vi "Init.vi"(8 "error in (no error)":errorcluster, 10 "Address":string, 11 "ArduinoTranslationStage in":refnum<class "ArduinoTranslationStage.lvclass">) -> (0 "error out":errorcluster, 3 "ArduinoTranslationStage out":refnum<class "ArduinoTranslationStage.lvclass">)   [LabVIEW 2023, in "ArduinoTranslationStage.lvlib" / "ArduinoTranslationStage.lvclass"]
uses:
  ArduinoTranslationStage.lvclass
  ArduinoTranslationStage.lvclass/ArduinoTranslationStage.ctl
  <vilib>/Instr/_visa.llb/Select Event Type.ctl
  Interfaces/InitDeinitInterface/InitDeinitComm Messages/InitDone Msg/InitDone Msg.lvclass
  <vilib>/ActorFramework/Actor/Actor.lvclass
  typedefs/instrumentType.ctl
  typedefs/typedefs.lvlib
  Applications/National Instruments/LabVIEW 2023 64-bit/vi.lib/ActorFramework/Actor/Actor.lvclass
  Users/alexandrosspiliotis/Documents/LV_DAQ_Project/UIs/ArduinoTranslationStageUI/ArduinoTranslationStageActor/ArduinoTranslationStage Actor/ArduinoTranslationStage.lvclass
  Users/alexandrosspiliotis/Documents/LV_DAQ_Project/Interfaces/InitDeinitInterface/InitDeinit/InitDeinit.lvclass
  Users/alexandrosspiliotis/Documents/LV_DAQ_Project/Interfaces/AbstractInstrumentClasses/StepperMotorControllers_LV/StepperMotorController/StepperMotorController.lvclass
  Users/alexandrosspiliotis/Documents/LV_DAQ_Project/Interfaces/AbstractInstrumentClasses/TranslationStages_LV/TranslationStageInterface/TranslationStagesInterface.lvclass
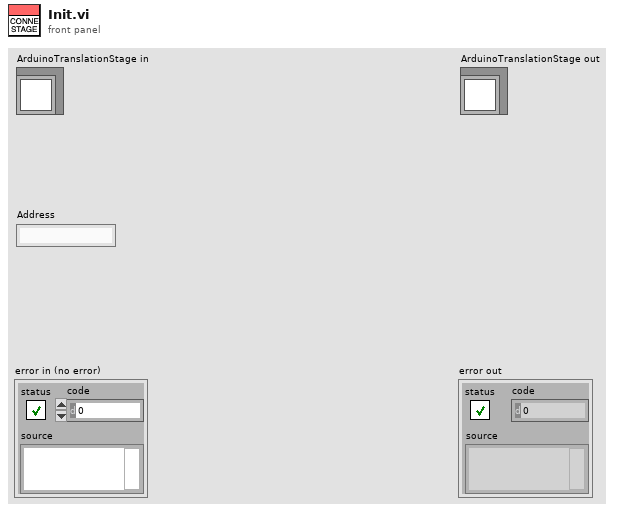
[diagram p1: front panel]
types:
  T1 = typedef "typedefs.lvlib/instrumentType.ctl" = enum16{"Spectrometer", "Camera", "Stepper"}
  T2 = typedef "Select Event Type.ctl" = u32
  T3 = typedef "typedefs.lvlib/InstrumentData.ctl" = cluster{"Instr Error":errorcluster, "Address":cluster{"address type":enum16{"VISA", "Index"}, "Address":string, "instrument type":T1}, "CurrentState":cluster{"Initialized":bool, "Connected":bool, "Running":bool, "Error":bool}, "Enqueuer":refnum<class "Message Enqueuer.lvclass">}
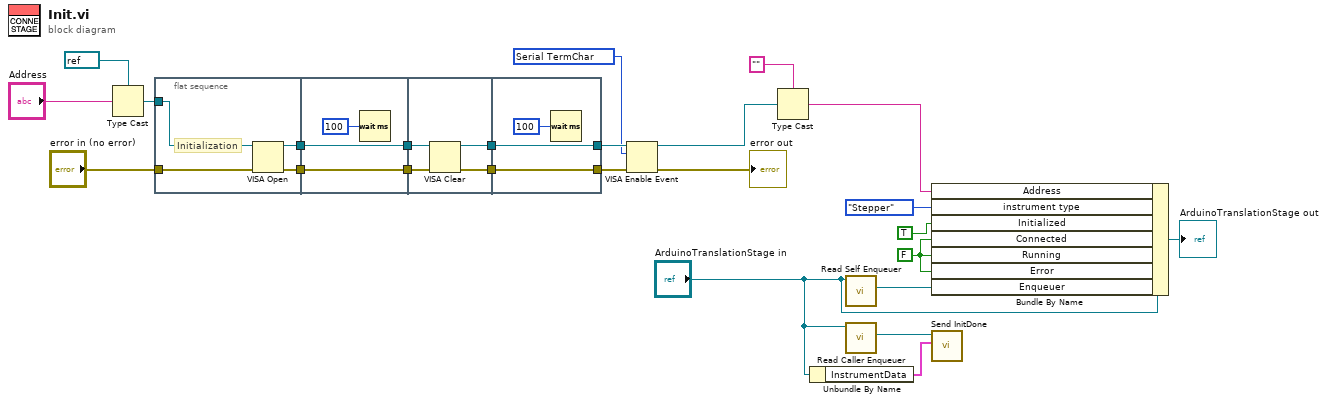
[diagram p0: block diagram]
diagram:
  w3 = FALSE ("InstrumentData.CurrentState.Connected")
  w17 = T2 1073684516 items=["Service Request"=1073684491, "Trigger"=3221168138, "Clear"=1073684493, "VXI Signal"=1073684512, "VXI/VME Interrupt"=3221168161, "VXI/VME Sysfail"=1073684509, "VXI/VME Sysreset"=1073684510, "GPIB CIC"=1073684498, "GPIB Talk"=1073684499, "GPIB Listen"=1073684500, "PXI Interrupt"=1073684514, "Serial Break"=1073684515, "Serial TermChar"=1073684516, "Serial CTS"=1073684521, "Serial DSR"=1073684522, "Serial DCD"=1073684524, "Serial RI"=1073684526, "Serial Character"=1073684533, "USB Interrupt"=1073684535, "All Enabled"=1073709055] ("Event Type")
  n1 = Type Cast(type=refnum<visa-resource-name> refnum ("VISA resource name"), x="Address") -> (*(type *) &x=w14:refnum<visa-resource-name>)
  n2 = flat-sequence {
    tunnel: [w29] -> w25
    tunnel: [w28] -> w24
    tunnel: w14 -> [w27]
    tunnel: "error in (no error)" -> [w26]
    tunnel: [w31] -> w23
    tunnel: w25 -> [w31]
    tunnel: [w30] -> w22
    tunnel: w24 -> [w30]
    tunnel: [w34] -> w21
    tunnel: [w33] -> w20
    tunnel: w23 -> [w36]
    tunnel: w22 -> [w35]
    tunnel: [w38] -> w18
    tunnel: [w39] -> w19
    tunnel: w21 -> [w39]
    tunnel: w20 -> [w38]
    frame #0 {
      # "Initialization"
      n3 = VISA Open(error in (no error)=w26, VISA resource name=w27) -> (VISA resource name=w28:refnum<visa-resource-name>, error out=w29:errorcluster)  [unwired: 3 in]
    }
    frame #1 {
      n4 = Wait (ms)(milliseconds to wait=u32 100) -> ()  [unwired: 1 out]
    }
    frame #2 {
      n5 = VISA Clear(VISA resource name=w35, error in (no error)=w36) -> (VISA resource name out=w33:refnum<visa-resource-name>, error out=w34:errorcluster)
    }
    frame #3 {
      n6 = Wait (ms)(milliseconds to wait=u32 100) -> ()  [unwired: 1 out]
    }
  }
  n7 = VISA Enable Event(8:w19, 10:w17, 11:w18) -> (0:→"error out":errorcluster, 3:w8:refnum<visa-resource-name>)  [unwired: 1 in]
  n8 = Type Cast(type="", x=w8) -> (*(type *) &x=w7:string)
  n9 = Unbundle By Name("ArduinoTranslationStage in") -> ("InstrumentData"=w6:T3)
  n10 = call <vilib>:"Read Self Enqueuer.vi"("Actor"="ArduinoTranslationStage in") -> ("Self Enqueuer"=w1:refnum<class "Message Enqueuer.lvclass">)  [unwired: 10 in]
  n11 = call <vilib>:"Read Caller Enqueuer.vi"("Actor"="ArduinoTranslationStage in") -> ("Caller Enqueuer"=w11:refnum<class "Message Enqueuer.lvclass">)  [unwired: 10 in]
  n12 = Bundle By Name(cluster="ArduinoTranslationStage in", "Address"=w7, "instrument type"=instrumentType."Stepper" ("InstrumentData.Address.instrument type"), "Initialized"=TRUE ("InstrumentData.CurrentState.Initialized"), "Connected"=w3, "Running"=w3, "Error"=w3, "Enqueuer"=w1) -> (→"ArduinoTranslationStage out":refnum<class "ArduinoTranslationStage.lvclass">)
  n13 = call "Send InitDone.vi"("InstrumentData"=w6, "Message Enqueuer"=w11) -> ()  [unwired: 8 in, 2 out]
